vi "Set Image from Vi.vi"(6 "Button Style":T1=enum."Classic", 7 "Button Size":i32, 8 "error in (no error)":errorcluster, 9 "State":T2, 10 "VI Refnum":refnum<vi>, 11 "Button in":refnum<class "Button.lvclass">) -> (0 "error out":errorcluster, 3 "Button out":refnum<class "Button.lvclass">)   [LabVIEW 2018, in "Button.lvclass"]
uses:
  Button.lvclass
  Type Defs/Button Status.ctl
  Type Defs/Button Style.ctl
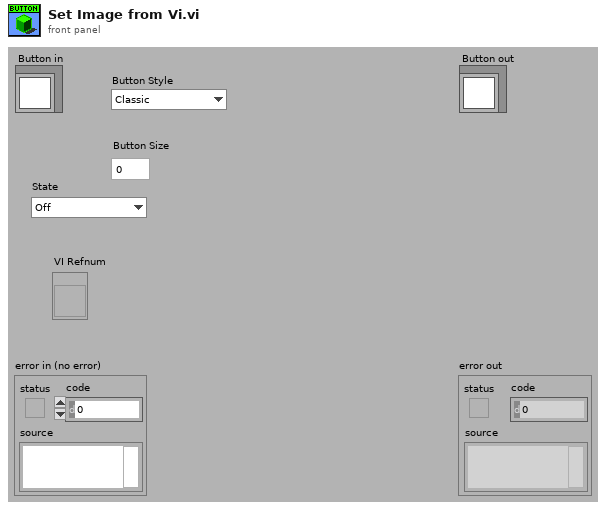
[diagram p1: front panel]
types:
  T1 = typedef "Button.lvclass/Button Style.ctl" = enum16{"System", "Modern", "Classic", "Rounded", "Silver", "Ni Theme", "Metallic"}
  T2 = typedef "Button.lvclass/Button Status.ctl" = enum16{"Off", "Hover", "On", "Disabled"}
  T3 = typedef "imagedata.ctl" = cluster{"image type":i32, "image depth":i32, "image":u8[], "mask":u8[], "colors":u32[], "Rectangle":cluster{"left":i16, "top":i16, "right":i16, "bottom":i16}}
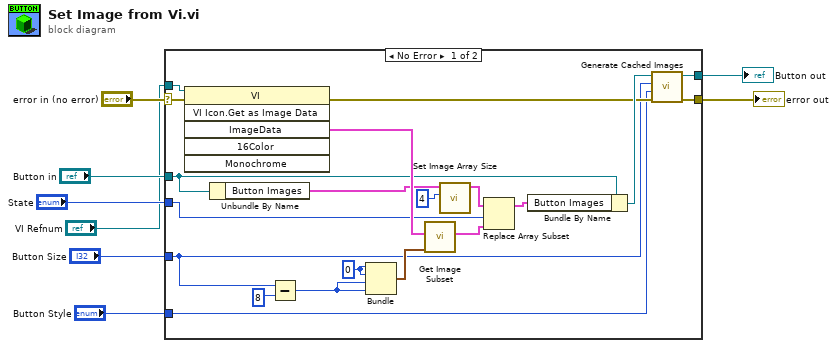
[diagram p0: block diagram]
diagram:
  n1 = case shown="No Error" "error in (no error)" {
    selector: "error in (no error)" -> [w19 w30]
    tunnel: [w11 w30] -> w7
    tunnel: [w13 w29] -> w5
    tunnel: "Button in" -> [w21 w29]
    tunnel: "State" -> [w22 _]
    tunnel: "VI Refnum" -> [w18 _]
    tunnel: "Button Size" -> [w10 _]
    tunnel: "Button Style" -> [w9 _]
    frame No Error {
      w26 = 0
      n2 = invoke class="VI" method="VI Icon.Get as Image Data"(reference=w18, error in=w19) -> (error out=w12:errorcluster, "ImageData"=w24:T3)  [unwired: 4 in, 4 out]
      n3 = Unbundle By Name(w21) -> ("Button Images"=w16:T3[])
      n4 = Subtract(x=w10, y=8) -> (x-y=w27:i32)
      n5 = Bundle(w26, w26, w27, w27) -> (w25:cluster{i32, i32, i32, i32})  [unwired: 1 out]
      n6 = call <vilib>:"Get Image Subset.vi"("subset rect"=w25, "image data"=w24) -> ("image subset"=w23:T3)  [unwired: 2 in, 3 out]
      n7 = call "Set Image Array Size.vi"("Buttons Displayed"=4, "Button Images in"=w16) -> ("Button Images out"=w14:T3[])  [unwired: 9 in]
      n8 = Replace Array Subset(array=w14, new element=w23, index=w22) -> (w15:T3[])
      n9 = Bundle By Name(cluster=w21, "Button Images"=w15) -> (w20:refnum<class "Button.lvclass">)
      n10 = call-dynamic "Generate Cached Images.vi"("error in (no error)"=w12, "Button Style"=w9, "Button Size"=w10, "object in"=w20) -> ("error out"=w11:errorcluster, "object out"=w13:refnum<class "Button.lvclass">)  [unwired: 6 in]
    }
    frame Error {
    }
  }
  "error out" <- w7
  "Button out" <- w5
